vi "Scroll Gradient.vi"(8 "error in (no error)":errorcluster caption="错误输入（无错误）", 11 "Scroll Gradient 输入":refnum<class "Scroll Gradient.lvclass"> caption="DNL_LabVIEW Object in") -> (0 "error out":errorcluster caption="错误输出", 3 "Scroll Gradient 输出":refnum<class "Scroll Gradient.lvclass"> caption="DNL_LabVIEW Object out")   [LabVIEW 2011, in "Scroll Gradient.lvclass"]
uses:
  Scroll Gradient.lvclass
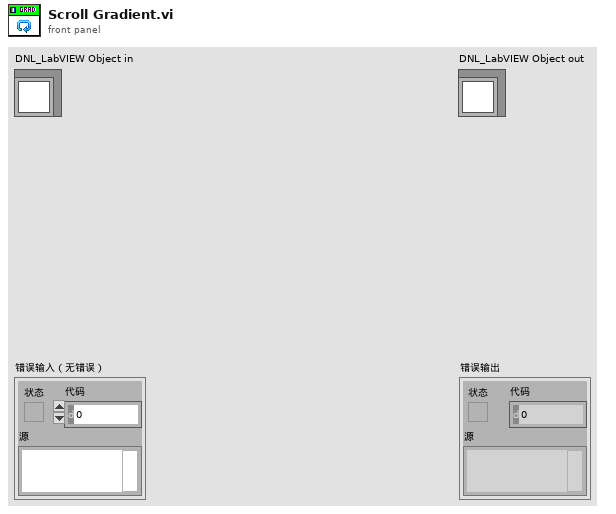
[diagram p1: front panel]
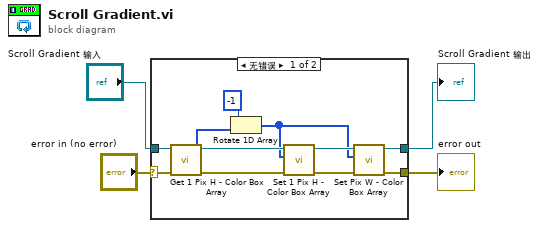
[diagram p0: block diagram]
diagram:
  n1 = case shown="无错误" "error in (no error)" {
    selector: "error in (no error)" -> [w14 w17]
    tunnel: [w8 w17] -> w3
    tunnel: [w9 w16] -> w1
    tunnel: "Scroll Gradient 输入" -> [w15 w16]
    frame No Error {
      n2 = call "Get 1 Pix H - Color Box Array.vi"("error in (no error)"=w14, "Scroll Gradient输入"=w15) -> ("error out"=w10:errorcluster, "1 Pix H - Color Box Array"=w13:u32[], "Scroll Gradient输出"=w11:refnum<class "Scroll Gradient.lvclass">)  [unwired: 7 in]
      n3 = Rotate 1D Array(1:w13, 2:-1 ("n")) -> (0:w6:u32[])
      n4 = call "Set 1 Pix H - Color Box Array.vi"("error in (no error)"=w10, "1 Pix H - Color Box Array"=w6, "Scroll Gradient输入"=w11) -> ("error out"=w5:errorcluster, "Scroll Gradient输出"=w7:refnum<class "Scroll Gradient.lvclass">)  [unwired: 7 in]
      n5 = call "Set Pix W - Color Box Array.vi"("error in (no error)"=w5, "1 Pix W - Color Box Array"=w6, "Scroll Gradient输入"=w7) -> ("error out"=w8:errorcluster, "Scroll Gradient输出"=w9:refnum<class "Scroll Gradient.lvclass">)  [unwired: 7 in]
    }
    frame Error {
    }
  }
  "error out" <- w3
  "Scroll Gradient 输出" <- w1
